vi "read revision fix.vi"(8 "error in":errorcluster, 11 "shared memory editor node":refnum<class "module editor node.lvclass">) -> (0 "error out":errorcluster, 2 "revision fix":u16, 3 "shared memory editor node out":refnum<class "module editor node.lvclass">)   [LabVIEW 2013, in "Shared Memory editor node.lvclass"]
uses:
  Shared Memory editor node.lvclass
  <vilib>/NI/DCAF/Tag Editor Core/Configuration Editor/Classes/Module editor node/module editor node.lvclass
  module/configuration/Shared Memory configuration.lvclass
  <vilib>/NI/Configuration Framework/serializable configuration/NISE_CEF_serializable configuration.lvclass
  module/configuration/Shared Memory configuration.lvclass/Shared Memory configuration.ctl
  module/configuration/Read revision fix.vi
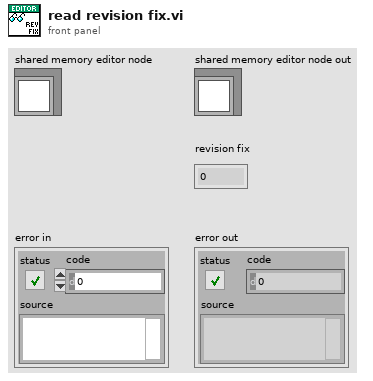
[diagram p1: front panel]
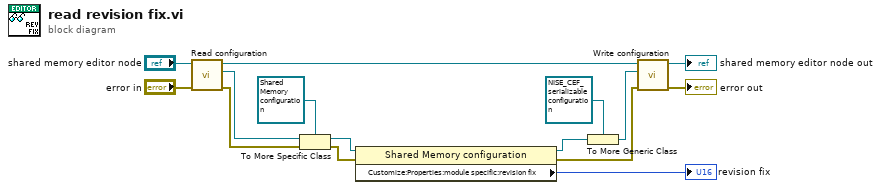
[diagram p0: block diagram]
diagram:
  n1 = call-dynamic "Read configuration.vi"("error in"="error in", "NISE_CEF_serializable node in"="shared memory editor node") -> ("error out"=w12:errorcluster, "configuration"=w13:refnum<class "NISE_CEF_serializable configuration.lvclass">, "NISE_CEF_serializable node out"=w6:refnum<class "module editor node.lvclass">)  [unwired: 7 in]
  n2 = To More Specific Class(target class=refnum<class "Shared Memory configuration.lvclass"> refnum ("shared memory configuration"), reference=w13, error in=w12) -> (specific class reference=w11:refnum<class "Shared Memory configuration.lvclass">, error out=w10:errorcluster)
  n3 = property class="Shared Memory configuration"(reference=w11, error in=w10) -> (reference out=w9:refnum<class "Shared Memory configuration.lvclass">, error out=w5:errorcluster, "Customize:Properties:module specific:revision fix"=→"revision fix":u16)
  n4 = To More Generic Class(target class=refnum<class "NISE_CEF_serializable configuration.lvclass"> refnum ("configuration"), reference=w9) -> (generic class reference=w7:refnum<class "NISE_CEF_serializable configuration.lvclass">)
  n5 = call-dynamic "Write configuration.vi"("error in"=w5, "configuration"=w7, "NISE_CEF_serializable node in"=w6) -> ("error out"=→"error out":errorcluster, "NISE_CEF_serializable node out"=→"shared memory editor node out":refnum<class "module editor node.lvclass">)  [unwired: 7 in]
